vi "Populate_Do.vi"(8 "error in (no error)":errorcluster, 9 "Value":string, 10 "Lower case name":string, 11 "Action Interface in":refnum<class "Action Interface.lvclass">) -> (0 "error out":errorcluster, 1 "Success?":bool, 3 "Action Interface out":refnum<class "Action Interface.lvclass">)   [LabVIEW 2020, in "ProjectBuilder.lvlib" / "Action Interface.lvclass"]
doc: "Override to populate private data from strings.\n\nThe default implementation does nothing but return 'Success?'=True."
uses:
  Action Interface.lvclass
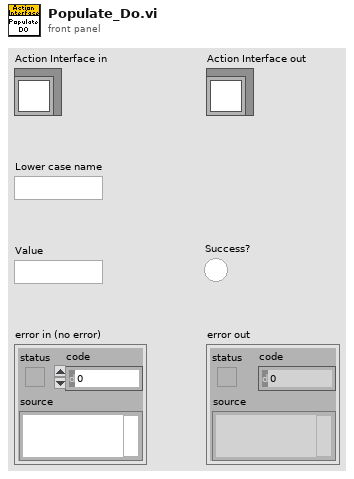
[diagram p1: front panel]
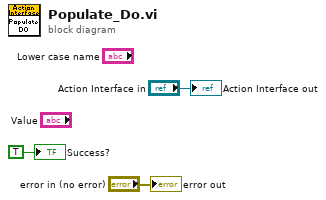
[diagram p0: block diagram]
diagram:
  "error out" <- "error in (no error)"
  "Action Interface out" <- "Action Interface in"
  "Success?" <- TRUE
